vi "DSF.Engine.Transfer Group.Is Active.vi"(10 "cycle count":u64=1, 11 "Transfer Group in":refnum<class "DSF.Engine.Transfer Group.lvclass">) -> (2 "active this cycle?":bool, 3 "Transfer Group out":refnum<class "DSF.Engine.Transfer Group.lvclass">)   [LabVIEW 2017, in "DSF.Engine.lvlib" / "DSF.Engine.Transfer Group.lvclass"]
uses:
  DSF.Engine.Transfer Group.lvclass
  DSF.Engine.Transfer Group.lvclass/DSF.Engine.Transfer Group.ctl
  Timing/DSF.Engine.Timing.lvclass/DSF.Engine.Timing.ctl
  Timing/DSF.Engine.Timing.Get Decimation.vi
  Timing/DSF.Engine.Timing.Get Offset.vi
  Timing/DSF.Engine.Timing.lvclass
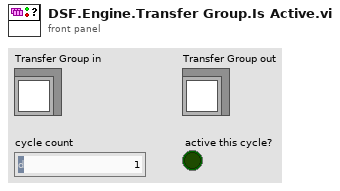
[diagram p1: front panel]
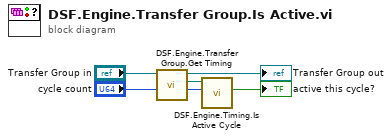
[diagram p0: block diagram]
diagram:
  n1 = call "DSF.Engine.Transfer Group.Get Timing.vi"("Transfer Group in"="Transfer Group in") -> ("Timing"=w4:refnum<class "DSF.Engine.Timing.lvclass">, "Transfer Group out"=→"Transfer Group out":refnum<class "DSF.Engine.Transfer Group.lvclass">)  [unwired: 9 in]
  n2 = call "DSF.Engine.Timing.Is Active Cycle.vi"("iteration"="cycle count", "Timing in"=w4) -> ("active?"=→"active this cycle?":bool)  [unwired: 8 in, 1 out]
